vi "Untitled 1.vi"   [LabVIEW 2014]
uses:
  ADDI-DATA MSX-E3701/API/Typedef/Diagnostic Data.ctl
  ADDI-DATA MSX-E3701/API/MSX-E3701_dll.lvlib
types:
  T1 = typedef "MSX-E3701_dll.lvlib/Diagnostic Data.ctl" = cluster{"Muestras Diag. Cycle":u32, "Tolerancia Cycle":sgl, "Tolerancia":sgl, "Mask Proteccion T":u64, "Promedio Transd":sgl[]}
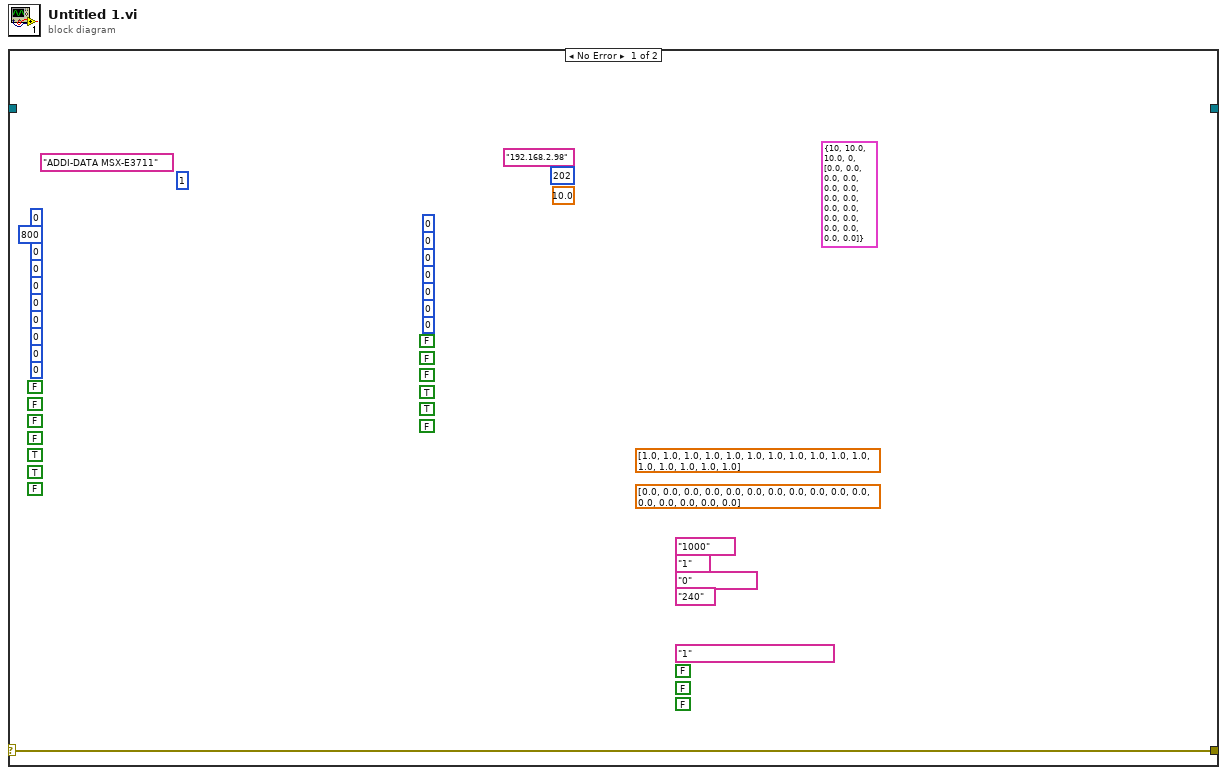
[diagram p0: block diagram]
diagram:
  n1 = case shown="No Error" {
    selector: _ -> [w49 w51]
    tunnel: [w49 w51] -> _
    tunnel: [w9 w50] -> _
    tunnel: _ -> [w38 w50]
    frame No Error {
      w1 = "240" ("FrequencySelection")
      w2 = "0" ("InitGainSelection")
      w3 = "1" ("ConvertMode")
      w4 = "1000" ("ConnectedTempSensor")
      w6 = FALSE ("CounterClear")
      w5 = FALSE ("CounterOptionOthers")
      w8 = FALSE ("CounterOptionDIRECT")
      w7 = "1" ("CounterMode")
      w16 = u64 0 ("Config Data.Auto Refresh.By Trigger Nbr Of Seq To Acquire")
      w19 = FALSE ("Config Data.Auto Refresh.Invert value")
      w18 = FALSE ("Config Data.Auto Refresh.Analog Output(mm)")
      w17 = FALSE ("Config Data.Auto Refresh.Time stamp")
      w23 = u64 0 ("Config Data.Sequence.By Trigger Nbr Of Seq To Acquire")
      w31 = FALSE ("Config Data.Sequence.Time stamp")
      w14 = u64 0 ("Config Data.Auto Refresh.Average Value")
      w39 = T1 {"Muestras Diag. Cycle"=10, "Tolerancia Cycle"=10.0, "Tolerancia"=10.0, "Mask Proteccion T"=0, "Promedio Transd"=[0.0, 0.0, 0.0, 0.0, 0.0, 0.0, 0.0, 0.0, 0.0, 0.0, 0.0, 0.0, 0.0, 0.0, 0.0, 0.0]} ("Diagnostic Data")
      w40 = sgl 10.0 ("Config Data.Range")
      w41 = u64 202 ("Config Data.Index")
      w42 = "192.168.2.98" ("Connection Data.IP")
      w43 = sgl[] [0.0, 0.0, 0.0, 0.0, 0.0, 0.0, 0.0, 0.0, 0.0, 0.0, 0.0, 0.0, 0.0, 0.0, 0.0, 0.0] ("Config Data.Offset")
      w44 = sgl[] [1.0, 1.0, 1.0, 1.0, 1.0, 1.0, 1.0, 1.0, 1.0, 1.0, 1.0, 1.0, 1.0, 1.0, 1.0, 1.0] ("Config Data.Gain")
      w37 = FALSE ("Config Data.Sequence.Hardware trigger information")
      w36 = TRUE ("Config Data.Sequence.Relative Time Stamp")
      w35 = TRUE ("Config Data.Sequence.Invert value")
      w34 = FALSE ("Config Data.Sequence.Analog Output(mm)")
      w33 = FALSE ("Config Data.Sequence.Sequence counter information")
      w32 = FALSE ("Config Data.Sequence.Time stamp")
      w24 = u64 0 ("Config Data.Sequence.By Trigger Nbr Of Seq To Acquire")
      w25 = u64 0 ("Config Data.Sequence.Hardware Trigger Filter Time")
      w26 = u64 0 ("Config Data.Sequence.Hardware Trigger Count")
      w27 = u64 0 ("Config Data.Sequence.Trigger Action")
      w28 = u64 0 ("Config Data.Sequence.Delay Value")
      w29 = u64 0 ("Config Data.Sequence.Delay Time Unit")
      w30 = u64 0 ("Config Data.Sequence.Delay Mode")
      w45 = u64 800 ("Config Data.Sequence.Nbr Max Sequence To Transfer")
      w46 = u64 0 ("Config Data.Sequence.Nbr Of Sequence")
      w22 = FALSE ("Config Data.Auto Refresh.Invert value")
      w21 = TRUE ("Config Data.Auto Refresh.Analog Output(mm)")
      w20 = TRUE ("Config Data.Auto Refresh.Time stamp")
      w10 = u64 0 ("Config Data.Auto Refresh.By Trigger Nbr Of Seq To Acquire")
      w11 = u64 0 ("Config Data.Auto Refresh.Hardware Trigger Filter Time")
      w15 = u64 0 ("Config Data.Auto Refresh.Hardware Trigger Count")
      w12 = u64 0 ("Config Data.Auto Refresh.Trigger Action")
      w13 = u64 0 ("Config Data.Auto Refresh.Average Value")
      w47 = u64 1 ("Channel Mask")
      w48 = "ADDI-DATA MSX-E3711" ("Driver Name")
    }
    frame Error {
    }
  }
